vi "PH_PP_CurrentMeas_Startup.vi"   [LabVIEW 2009]
panel:
  # "This is the StartupVI of the RT Application for the PHELIX PPMA DAQ.\n\nEach of the identical VIs starts a Listener with a unique port for each DAQ Module.\n\nFor the moment this VI has to be downloaded and started from the \nLVRT develeopment system after power on once. The VI is programmed to run forever!"
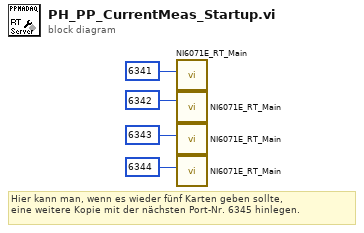
[diagram p0: block diagram]
diagram:
  # "Hier kann man, wenn es wieder fünf Karten geben sollte,\neine weitere Kopie mit der nächsten Port-Nr. 6345 hinlegen."
  n1 = call "NI6071E_RT_Main.vi"("Port"=u16 6341) -> ()  [unwired: 10 in]
  n2 = call "NI6071E_RT_Main.vi"("Port"=u16 6342) -> ()  [unwired: 10 in]
  n3 = call "NI6071E_RT_Main.vi"("Port"=u16 6343) -> ()  [unwired: 10 in]
  n4 = call "NI6071E_RT_Main.vi"("Port"=u16 6344) -> ()  [unwired: 10 in]
